vi "Practica2Ejercicio1.vi"() -> ()   [LabVIEW 2014]
uses:
  <vilib>/MakerHub/LINX/Public/Peripherals/Analog/Analog Read 1 Chan.vi
  <vilib>/MakerHub/LINX/Public/Peripherals/Digital/Digital Write 1 Chan.vi
  <vilib>/MakerHub/LINX/Public/Peripherals/Analog/Analog Read N Chans.vi
  <vilib>/MakerHub/LINX/Public/Peripherals/Digital/Digital Write N Chans.vi
  <vilib>/MakerHub/LINX/Private/Local IO/LinxAnalogRead.vi
  <vilib>/MakerHub/LINX/Public/Utilities/Check Channel.vi
  <vilib>/MakerHub/LINX/Private/Local IO/LinxDigitalWrite.vi
  <vilib>/MakerHub/LINX/Public/Utilities/Open Serial.vi
  <vilib>/MakerHub/LINX/Private/Utilties/Generate Error.vi
  <vilib>/MakerHub/LINX/LMH-LINX.lvlib
panel:
  out "Boolean 2":bool
  out "Boolean":bool
  in  "Stop Button":bool
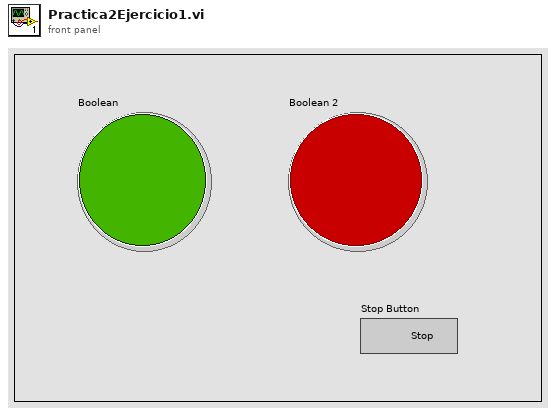
[diagram p1: front panel]
types:
  T1 = typedef "LMH-LINX.lvlib/LINX Ref.ctl" = cluster{"IO":T2, "Interface":T3, "LINX Device Config":T4}
  T2 = typedef "LMH-LINX.lvlib/Platform.ctl" = enum16{"Remote", "Local"}
  T3 = typedef "LMH-LINX.lvlib/Interface.ctl" = enum16{"Serial", "TCP"}
  T4 = typedef "LMH-LINX.lvlib/Device.lvlib/LINX Device Config.ctl" = cluster{"Interface":T3, "COM Port":refnum<visa-resource-name>, "TCP Configuration":T5, "Device Family":u8, "Device ID":u8, "Device Name":string, "TCP Ref":refnum<k5>, "Channels":T6}
  T5 = typedef "LMH-LINX.lvlib/Device.lvlib/TCP Config.ctl" = cluster{"IP Address":string, "Port":u16}
  T6 = typedef "LMH-LINX.lvlib/Channels.ctl" = cluster{"DI":u8[], "DO":u8[], "AI":u8[], "AO":u8[], "PWM":u8[], "QE":u8[], "UART":u8[], "I2C 2":u8[], "SPI":u8[], "CAN":u8[], "Servo":u8[], "AI Ref (V)":dbl, "AI Resolution (Bits)":u8, "AO Ref (V)":dbl, "AO Resolution (Bits)":u8}
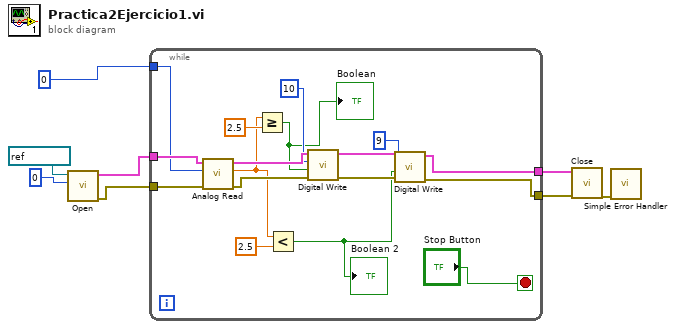
[diagram p0: block diagram]
diagram:
  n1 = call-poly <vilib>:"Open.vi"("Baud Rate Override"=u32 0, "Serial Port"=refnum<visa-resource-name> "COM5") -> ("Error Out"=w7:errorcluster, "LINX Resource"=w8:T1)  [unwired: 7 in, 1 out]
  n2 = while {
    tunnel: w8 -> [w25]
    tunnel: w7 -> [w24]
    tunnel: u8 0 ("Analog Input Pin (0)") -> [w22]
    tunnel: [w12] -> w2
    tunnel: [w11] -> w1
    stop <- "Stop Button" stop-if-true
    n3 = call-poly <vilib>:"Analog Read.vi"("Error In"=w24, "Analog Channel"=w22, "LINX Resource"=w25) -> ("Error Out"=w19:errorcluster, "Voltage"=w14:dbl, "LINX Resource"=w20:T1)  [unwired: 5 in, 1 out]
    n4 = Greater Or Equal?(x=w14, y=2.5) -> (x >= y?=w10:bool)
    "Boolean" <- w10
    n5 = Less?(x=w14, y=2.5) -> (x < y?=w9:bool)
    "Boolean 2" <- w9
    n6 = call-poly <vilib>:"Digital Write.vi"("Error In"=w19, "Output Value"=w10, "DO Channel"=u8 10, "LINX Resource"=w20) -> ("Error Out"=w16:errorcluster, "LINX Resource"=w17:T1)  [unwired: 6 in]
    n7 = call-poly <vilib>:"Digital Write.vi"("Error In"=w16, "Output Value"=w9, "DO Channel"=u8 9, "LINX Resource"=w17) -> ("Error Out"=w11:errorcluster, "LINX Resource"=w12:T1)  [unwired: 6 in]
  }
  n8 = call <vilib>:"Close.vi"("Error In"=w1, "LINX Resource"=w2) -> ("Error Out"=w3:errorcluster)  [unwired: 9 in]
  n9 = call <vilib>:"Simple Error Handler.vi"("error in (no error)"=w3) -> ()  [unwired: 4 in, 5 out]
